vi "ExitNowAllLoops vxm.vi"(8 "error in (no error)":errorcluster, 11 "MessageQues":T1) -> (0 "error out":errorcluster)   [LabVIEW 2017]
doc: "Send ExitNow message to all loops.\n\n Execute all que operations even if there is an error in.\n\nBolder Software LLC"
uses:
  MultipleMessageQues vxm.ctl
  MessageQue.ctl
  MessageCluster.ctl
  MessageQue.lvlib
panel:
  # "SaveData Ques\nDisplay Que\nDisplayNotifier"
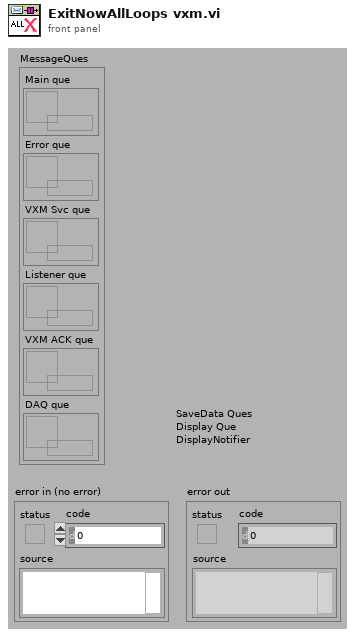
[diagram p1: front panel]
types:
  T1 = typedef "MultipleMessageQues vxm.ctl" = cluster{"Main que":T2, "Error que":T2, "VXM Svc que":T2, "Listener que":T2, "VXM ACK que":T2, "DAQ que":T2}
  T2 = typedef "MessageQue.lvlib/MessageQue.ctl" = refnum<queue>
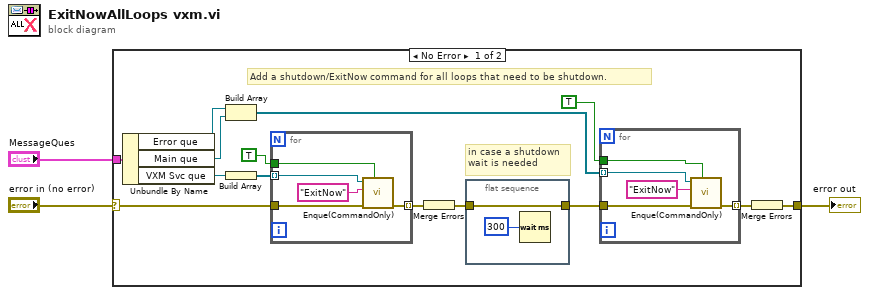
[diagram p0: block diagram]
diagram:
  n1 = case shown="No Error" "error in (no error)" {
    selector: "error in (no error)" -> [w17 w30]
    tunnel: [w10 w30] -> w2
    tunnel: "MessageQues" -> [w14 _]
    frame No Error {
      # "Add a shutdown/ExitNow command for all loops that need to be shutdown."
      # "in case a shutdown\nwait is needed"
      n2 = Unbundle By Name(w14) -> ("Error que"=w5:T2, "Main que"=w4:T2, "VXM Svc que"=w12:T2)
      n3 = Build Array(w5, w4) -> (w8:T2[])
      n4 = Build Array(w12) -> (w13:T2[])
      n5 = for {
        tunnel: w17 -> [w29]
        tunnel: TRUE ("at front (F)") -> [w25]
        tunnel: [w28] -> w15 mode=indexing
        tunnel: w13 -> [w26] mode=indexing
        n6 = call "Enque(CommandOnly).vi"("at front (F)"=w25, "error in"=w29, "Message Command"="ExitNow" ("Command"), "Message que"=w26) -> ("error out"=w28:errorcluster)  [unwired: 6 in, 1 out]
      }
      n7 = Merge Errors(w15) -> (w7:errorcluster)
      n8 = flat-sequence {
        tunnel: [w18] -> w6
        tunnel: w7 -> [w18]
        frame #0 {
          n9 = Wait (ms)(milliseconds to wait=u32 300) -> ()  [unwired: 1 out]
        }
      }
      n10 = for {
        tunnel: w6 -> [w23]
        tunnel: TRUE ("at front (F)") -> [w21]
        tunnel: [w22] -> w11 mode=indexing
        tunnel: w8 -> [w20] mode=indexing
        n11 = call "Enque(CommandOnly).vi"("at front (F)"=w21, "error in"=w23, "Message Command"="ExitNow" ("Command"), "Message que"=w20) -> ("error out"=w22:errorcluster)  [unwired: 6 in, 1 out]
      }
      n12 = Merge Errors(w11) -> (w10:errorcluster)
    }
    frame Error {
    }
  }
  "error out" <- w2
